vi "Create User Event - Stop.vi"(8 "error in (no error)":cluster{"状态":bool, "代码":i32, "源":string} caption="错误输入（无错误）") -> (0 "error out":cluster{"状态":bool, "代码":i32, "源":string} caption="错误输出", 3 "用户事件－停止":refnum<user-event>)   [LabVIEW 2025, in "User Event - Stop.lvlib"]
doc: "创建一个布尔用户事件，用于通过“消息处理循环”使“事件循环”停止执行。"
uses:
  User Event - Stop.lvlib
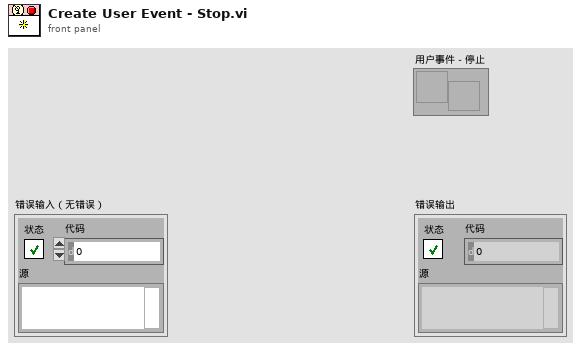
[diagram p1: front panel]
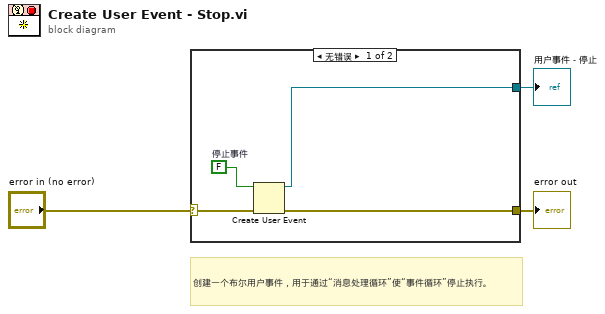
[diagram p0: block diagram]
diagram:
  # "创建一个布尔用户事件，用于通过“消息处理循环”使“事件循环”停止执行。"
  n1 = case shown="无错误" "error in (no error)" {
    selector: "error in (no error)" -> [w4 w8]
    tunnel: [w7 _] -> w3
    tunnel: [w5 w8] -> w2
    frame No Error {
      w6 = FALSE  # 停止事件
      n2 = Create User Event(user event datatype=w6, error in=w4) -> (user event=w7:refnum<user-event>, error out=w5:errorcluster)
    }
    frame Error {
    }
  }
  "用户事件－停止" <- w3
  "error out" <- w2
